vi "ELVIS III v1.0 Check For Different Banks.vi"(8 "error in (no error)":errorcluster, 11 "Channel Names":string[](array[string])) -> (0 "error out":errorcluster)   [LabVIEW 2021]
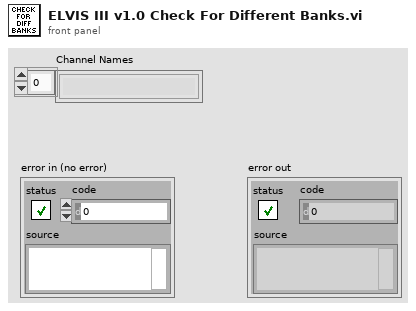
[diagram p1: front panel]
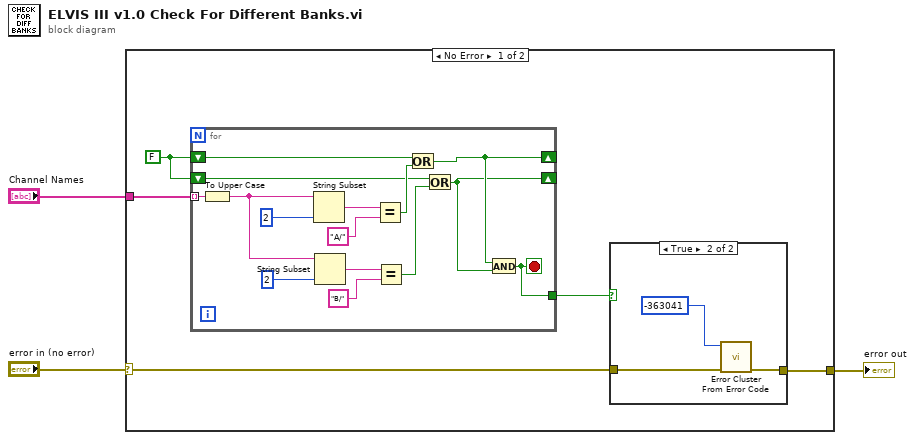
[diagram p0: block diagram]
diagram:
  n1 = case shown="No Error" "error in (no error)" {
    selector: "error in (no error)" -> [w6 w28]
    tunnel: "Channel Names" -> [w8 _]
    tunnel: [w5 w28] -> w1
    frame No Error {
      w7 = FALSE
      n2 = for {
        tunnel: w8 -> [w14] mode=indexing
        shift-right: [w15] -> _
        shift-left: w7 -> [w18]
        shift-right: [w16] -> _
        shift-left: w7 -> [w21]
        tunnel: [w17] -> w4
        stop <- w17 stop-if-true
        n3 = To Upper Case(1:w14) -> (0:w13:string)
        n4 = String Subset(string=w13, length (rest)=2 ("length (rest)")) -> (substring=w26:string)  [unwired: 1 in]
        n5 = String Subset(string=w13, length (rest)=2 ("length (rest)")) -> (substring=w23:string)  [unwired: 1 in]
        n6 = Equal?(x=w26, y="A/") -> (x = y?=w20:bool)
        n7 = Equal?(x=w23, y="B/") -> (x = y?=w19:bool)
        n8 = Or(x=w21, y=w20) -> (x .or. y?=w16:bool)
        n9 = Or(x=w18, y=w19) -> (x .or. y?=w15:bool)
        n10 = And(x=w16, y=w15) -> (x .and. y?=w17:bool)
      }
      n11 = case shown="True" w4 {
        tunnel: w6 -> [w9 w11]
        tunnel: [w9 w10] -> w5
        frame False {
        }
        frame True {
          n12 = call <vilib>:"Error Cluster From Error Code.vi"("error in (no error)"=w11, "error code (0)"=-363041) -> ("error out"=w10:errorcluster)  [unwired: 7 in]
        }
      }
    }
    frame Error {
    }
  }
  "error out" <- w1
